vi "Username.vi"(8 "error in":errorcluster) -> (0 "error out":errorcluster, 2 "Report Store Path_Out":path, 3 "User Name_Out":string)   [LabVIEW 2021]
doc: "Gets the Username"
uses:
  <vilib>/Utility/miscctls.llb/LVPointTypeDef.ctl
panel:
  in  "Report Store Path":path
  in  "Ok":bool
  in  "User Name":string
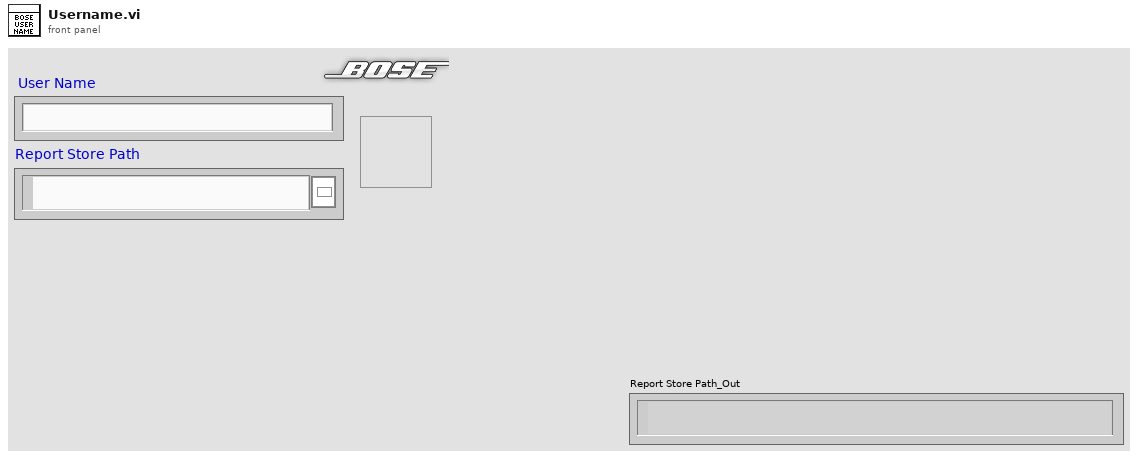
[diagram p1: front panel]
types:
  T1 = typedef "LVPointTypeDef.ctl" = cluster{"Horizontal":i16, "Vertical":i16}
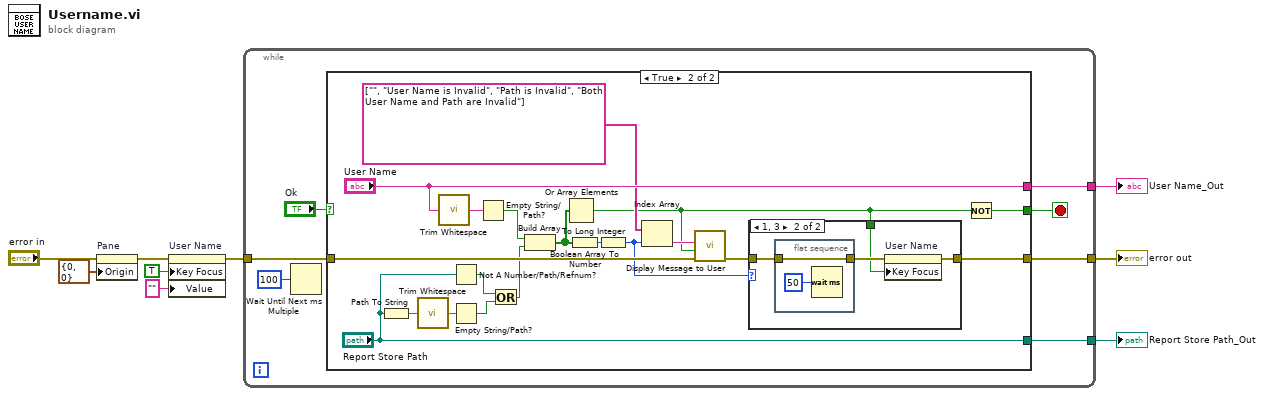
[diagram p0: block diagram]
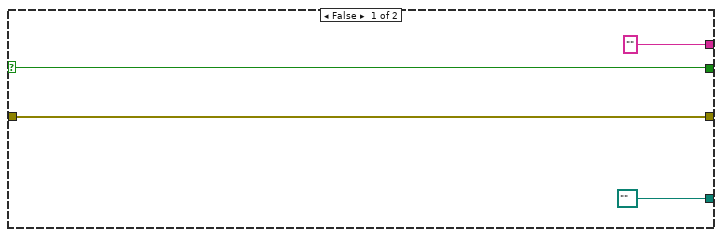
[diagram p2: hidden frame]
diagram:
  n1 = property on="Pane" class="Pane"(error in="error in", "Origin"=T1 {"Horizontal"=0, "Vertical"=0}) -> (error out=w6:errorcluster)  [unwired: 1 in, 1 out]
  n2 = property on="User Name" class="Str"(error in=w6, "Key Focus"=TRUE, "Value"="" ("User Name")) -> (error out=w5:errorcluster)  [unwired: 1 in, 1 out]
  n3 = while {
    tunnel: w5 -> [w14]
    tunnel: [w13] -> w1
    tunnel: [w11] -> w3
    tunnel: [w10] -> w2
    stop <- w15 stop-if-true
    n4 = Wait Until Next ms Multiple(millisecond multiple=u32 100) -> ()  [unwired: 1 out]
    n5 = case shown="True" "Ok" {
      selector: "Ok" -> [w20 _]
      tunnel: [w20 w35] -> w15
      tunnel: w14 -> [w19 w38]
      tunnel: [w19 w37] -> w13
      tunnel: ["" ("User Name") "User Name"] -> w11
      tunnel: [path "" ("Report Store Path") "Report Store Path"] -> w10
      frame False {
      }
      frame True {
        n6 = Path To String(path="Report Store Path") -> (string=w22:string)
        n7 = call <vilib>:"Trim Whitespace.vi"("string"=w22) -> ("trimmed string"=w21:string)  [unwired: 1 in]
        n8 = call <vilib>:"Trim Whitespace.vi"("string"="User Name") -> ("trimmed string"=w39:string)  [unwired: 1 in]
        n9 = Not A Number/Path/Refnum?(number/path/refnum="Report Store Path") -> (NaN/Path/Refnum?=w25:bool)
        n10 = Empty String/Path?(string/path=w21) -> (empty?=w24:bool)
        n11 = Empty String/Path?(string/path=w39) -> (empty?=w33:bool)
        n12 = Or(x=w25, y=w24) -> (x .or. y?=w23:bool)
        n13 = Build Array(w33, w23) -> (w28:bool[])
        n14 = Or Array Elements(Boolean array=w28) -> (logical OR=w27:bool)
        n15 = Boolean Array To Number(Boolean array=w28) -> (number=w31:u32)
        n16 = To Long Integer(number=w31) -> (32bit integer=w29:i32)
        n17 = Index Array(array=string[] ["", "User Name is Invalid", "Path is Invalid", "Both User Name and Path are Invalid"], index=w29) -> (element=w30:string)
        n18 = call "Display Message to User"("error in (no error)"=w38, "Enable"=w27, "Message"=w30) -> ("error out"=w36:errorcluster)  [unwired: 7 in, 1 out]
        n19 = case shown="1, 3" w29 {
          tunnel: [w40 w44] -> w37
          tunnel: w36 -> [w40 w43]
          tunnel: w27 -> [_ w41]
          frame 0, Default {
          }
          frame 1, 3 {
            n20 = flat-sequence {
              tunnel: w43 -> [w46]
              tunnel: [w46] -> w42
              frame #0 {
                n21 = Wait (ms)(milliseconds to wait=u32 50) -> ()  [unwired: 1 out]
              }
            }
            n22 = property on="User Name" class="Str"(error in=w42, "Key Focus"=w41) -> (error out=w44:errorcluster)  [unwired: 1 in, 1 out]
          }
        }
        n23 = Not(x=w27) -> (.not. x?=w35:bool)
      }
    }
  }
  "error out" <- w1
  "User Name_Out" <- w3
  "Report Store Path_Out" <- w2
